vi "发送数据记录到文档(子VI).vi"(7 "错误输入":errorcluster, 9 "字符串":string="报文记录", 10 "数组":string[](array[string])) -> (0 "错误输出":errorcluster)   [LabVIEW 2016, in "数据传输系统-04.lvlib"]
panel:
  out "路径":path
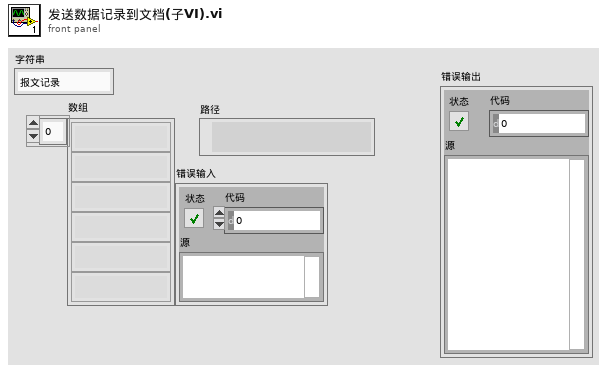
[diagram p1: front panel]
types:
  T1 = typedef "LVDateTimeRec.ctl" = cluster{"秒数的小数部分":dbl, "秒":i32, "分":i32, "时":i32, "日":i32, "月":i32, "年":i32, "天数（周）":i32, "天数（年）":i32, "DST":i32}
  T2 = enum16{"open", "replace", "create", "open or create", "replace or create", "replace or create with confirmation"}
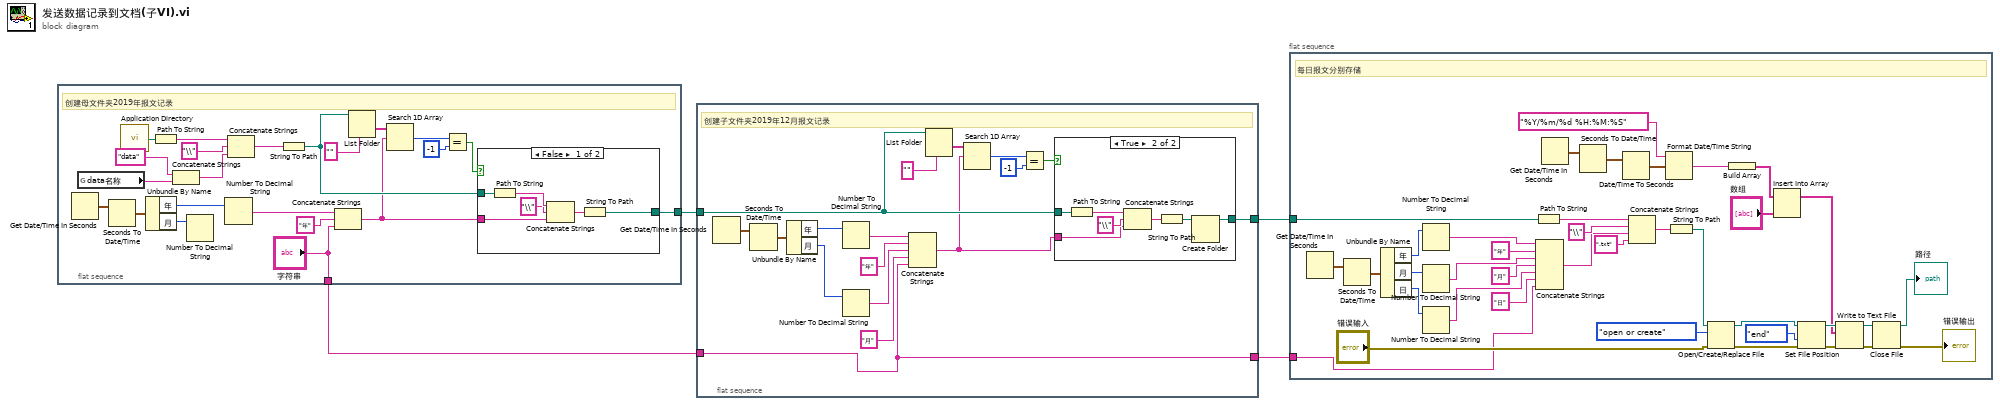
[diagram p0: block diagram]
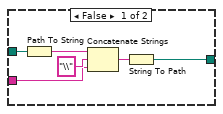
[diagram p2: hidden frame]
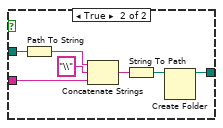
[diagram p3: hidden frame]
diagram:
  n1 = flat-sequence {
    tunnel: [w9] -> w4
    tunnel: ["字符串"] -> w2
    frame #0 {
      # "创建母文件夹2019年报文记录"
      n2 = Get Date/Time In Seconds() -> (seconds since 1Jan1904=w26:timestamp)
      n3 = global read "断电保存全局.vi" "data名称"() -> (w6:string)
      n4 = Seconds To Date/Time(time stamp (now)=w26) -> (date time rec=w25:T1)  [unwired: 1 in]
      n5 = call <vilib>:"Application Directory.vi"() -> ("Application Directory"=w14:path)
      n6 = Unbundle By Name(w25) -> ("年"=w24:i32, "月"=w23:i32)
      n7 = Path To String(path=w14) -> (string=w17:string)
      n8 = Concatenate Strings("data" ("名称或相对路径"), w6) -> (w5:string)
      n9 = Number To Decimal String(number=w23) -> ()  [unwired: 1 in, 1 out]
      n10 = Number To Decimal String(number=w24) -> (decimal integer string=w11:string)  [unwired: 1 in]
      n11 = Concatenate Strings(w17, "\\" ("字符串"), w5) -> (w15:string)
      n12 = String To Path(string=w15) -> (path=w13:path)
      n13 = Concatenate Strings(w11, "年" ("字符串"), "字符串") -> (w10:string)
      n14 = List Folder(path=w13, pattern="" ("类型")) -> (folder names=w18:string[])  [unwired: 2 in, 3 out]
      n15 = Search 1D Array(1D array=w18, element=w10) -> (index of element=w22:i32)  [unwired: 1 in]
      n16 = Equal?(x=w22, y=-1) -> (x = y?=w20:bool)
      n17 = case shown="False" w20 {
        tunnel: w13 -> [w30 w38]
        tunnel: w10 -> [w29 w35]
        tunnel: [w28 w39] -> w9
        frame False {
          n18 = Path To String(path=w30) -> (string=w32:string)
          n19 = Concatenate Strings(w32, "\\" ("字符串"), w29) -> (w27:string)
          n20 = String To Path(string=w27) -> (path=w28:path)
        }
        frame True {
          n21 = Path To String(path=w38) -> (string=w37:string)
          n22 = Concatenate Strings(w37, "\\" ("字符串"), w35) -> (w33:string)
          n23 = String To Path(string=w33) -> (path=w34:path)
          n24 = Create Folder(path (use dialog)=w34) -> (created path=w39:path)  [unwired: 2 in, 2 out]
        }
      }
    }
  }
  n25 = flat-sequence {
    tunnel: w4 -> [w43]
    tunnel: [w41] -> w3
    tunnel: w2 -> [w40]
    tunnel: [w40] -> w1
    frame #0 {
      # "创建子文件夹2019年12月报文记录"
      n26 = Get Date/Time In Seconds() -> (seconds since 1Jan1904=w46:timestamp)
      n27 = Seconds To Date/Time(time stamp (now)=w46) -> (date time rec=w47:T1)  [unwired: 1 in]
      n28 = Unbundle By Name(w47) -> ("年"=w48:i32, "月"=w49:i32)
      n29 = Number To Decimal String(number=w48) -> (decimal integer string=w51:string)  [unwired: 1 in]
      n30 = Number To Decimal String(number=w49) -> (decimal integer string=w45:string)  [unwired: 1 in]
      n31 = Concatenate Strings(w51, "年" ("字符串"), w45, "月" ("字符串"), w40) -> (w42:string)
      n32 = List Folder(path=w43, pattern="" ("类型")) -> (folder names=w56:string[])  [unwired: 2 in, 3 out]
      n33 = Search 1D Array(1D array=w56, element=w42) -> (index of element=w52:i32)  [unwired: 1 in]
      n34 = Equal?(x=w52, y=-1) -> (x = y?=w54:bool)
      n35 = case shown="True" w54 {
        tunnel: w43 -> [w59 w68]
        tunnel: w42 -> [w58 w65]
        tunnel: [w57 w69] -> w41
        frame False {
          n36 = Path To String(path=w59) -> (string=w62:string)
          n37 = Concatenate Strings(w62, "\\" ("字符串"), w58) -> (w60:string)
          n38 = String To Path(string=w60) -> (path=w57:path)
        }
        frame True {
          n39 = Path To String(path=w68) -> (string=w67:string)
          n40 = Concatenate Strings(w67, "\\" ("字符串"), w65) -> (w64:string)
          n41 = String To Path(string=w64) -> (path=w63:path)
          n42 = Create Folder(path (use dialog)=w63) -> (created path=w69:path)  [unwired: 2 in, 2 out]
        }
      }
    }
  }
  n43 = flat-sequence {
    tunnel: w3 -> [w81]
    tunnel: w1 -> [w70]
    frame #0 {
      # "每日报文分别存储"
      n44 = Get Date/Time In Seconds() -> (seconds since 1Jan1904=w105:timestamp)
      n45 = Seconds To Date/Time(time stamp (now)=w105) -> (date time rec=w104:T1)  [unwired: 1 in]
      n46 = Unbundle By Name(w104) -> ("年"=w103:i32, "月"=w102:i32, "日"=w99:i32)
      n47 = Number To Decimal String(number=w103) -> (decimal integer string=w100:string)  [unwired: 1 in]
      n48 = Number To Decimal String(number=w102) -> (decimal integer string=w106:string)  [unwired: 1 in]
      n49 = Number To Decimal String(number=w99) -> (decimal integer string=w97:string)  [unwired: 1 in]
      n50 = Path To String(path=w81) -> (string=w89:string)
      n51 = Concatenate Strings(w100, "年" ("字符串"), w106, "月" ("字符串"), w97, "日" ("字符串"), w70) -> (w83:string)
      n52 = Get Date/Time In Seconds() -> (seconds since 1Jan1904=w73:timestamp)
      n53 = Seconds To Date/Time(time stamp (now)=w73) -> (date time rec=w76:T1)  [unwired: 1 in]
      n54 = Date/Time To Seconds(2:w76) -> (0:w74:timestamp)  [unwired: 1 in]
      n55 = Concatenate Strings(w89, "\\" ("字符串"), w83, ".txt" ("字符串")) -> (w91:string)
      n56 = Format Date/Time String(time format string (%c)="%Y/%m/%d %H:%M:%S" ("时间格式字符串(%c)"), seconds (now)=w74) -> (date/time string=w77:string)  [unwired: 1 in]
      n57 = String To Path(string=w91) -> (path=w87:path)
      n58 = Open/Create/Replace File(file path (use dialog)=w87, error in="错误输入", operation (0:open)=T2."open or create" ("操作(0:open)")) -> (refnum out=w92:refnum<file>, error out=w93:errorcluster)  [unwired: 3 in, 1 out]
      n59 = Build Array(w77) -> (w72:string[])
      n60 = Insert Into Array(array=w72, new element="数组") -> (w71:string[])  [unwired: 1 in]
      n61 = Set File Position(refnum=w92, from (0:start)=enum16{"start", "end", "current"}."end" ("自（0:起始）"), error in=w93) -> (refnum out=w94:refnum<file>, error out=w95:errorcluster)  [unwired: 1 in]
      n62 = Write to Text File(file (use dialog)=w94, text=w71, error in=w95) -> (refnum out=w86:refnum<file>, error out=w85:errorcluster)  [unwired: 1 in, 1 out]
      n63 = Close File(refnum=w86, error in=w85) -> (path=→"路径":path, error out=→"错误输出":errorcluster)
    }
  }
